vi "WriteMessage.vi"(6 "Timeout(ms)":i32, 7 "Wait for Ack? (false)":bool, 8 "error in (no error)":errorcluster, 10 "Message":T1={"Command"="", "Arguments"=variant, " Msg Id"=-1}, 11 "NetworkConnection in":refnum<class "NetworkConnection.lvclass">) -> (0 "error out":errorcluster, 2 "StillConnected?":bool, 3 "NetworkConnection out":refnum<class "NetworkConnection.lvclass">, 4 "Timed Out?":bool)   [LabVIEW 2020, in "NetworkConnection.lvclass"]
doc: "Writes a message for the Remote System. The Wait Response? input indicates wheather this method sould wait for the remote system to send a receipt confirmation response or not.\n\nJKI Network Streams Connection 1.1.1.15\nJavier Ruiz - JKI\nCopyright (c) 2020, JKI\n\nThis library is provided \"AS IS\" ,WITHOUT WARRANTIES OR CONDITIONS OF ANY KIND, either express or implied."
uses:
  NetworkConnection.lvclass
  NetworkCommand--Cluster.ctl
  NetworkMessage--Cluster.ctl
  NetworkConnection.lvclass/NetworkConnection.ctl
  Clear Errors.vi
  Random Number Within Range - I32__ogtk.vi
  <resource>/objmgr/ni.dex.rc
panel:
  # "Copyright © 2020 JKI All rights reserved.\n\nAuthor: Javier Ruiz <javier.ruiz@jki.net>\n\nThis library is provided \"AS IS\" ,WITHOUT WARRANTIES OR \nCONDITIONS OF ANY KIND, either expressed or implied.\n\nJKI -- jki.net"
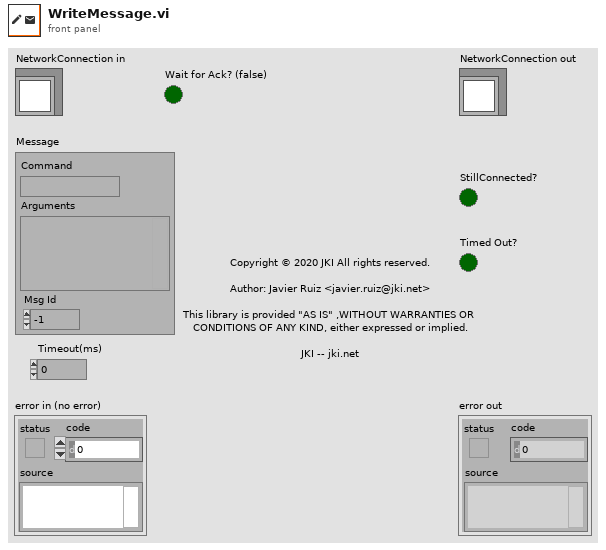
[diagram p1: front panel]
types:
  T1 = typedef "NetworkConnection.lvclass/NetworkCommand--Cluster.ctl" = cluster{"Command":string, "Arguments":variant, " Msg Id":i32}
  T2 = typedef "NetworkConnection.lvclass/NetworkMessage--Cluster.ctl" = cluster{"NetworkCommand":T1, "Wait for Ack?":bool, "Ack Id":i32}
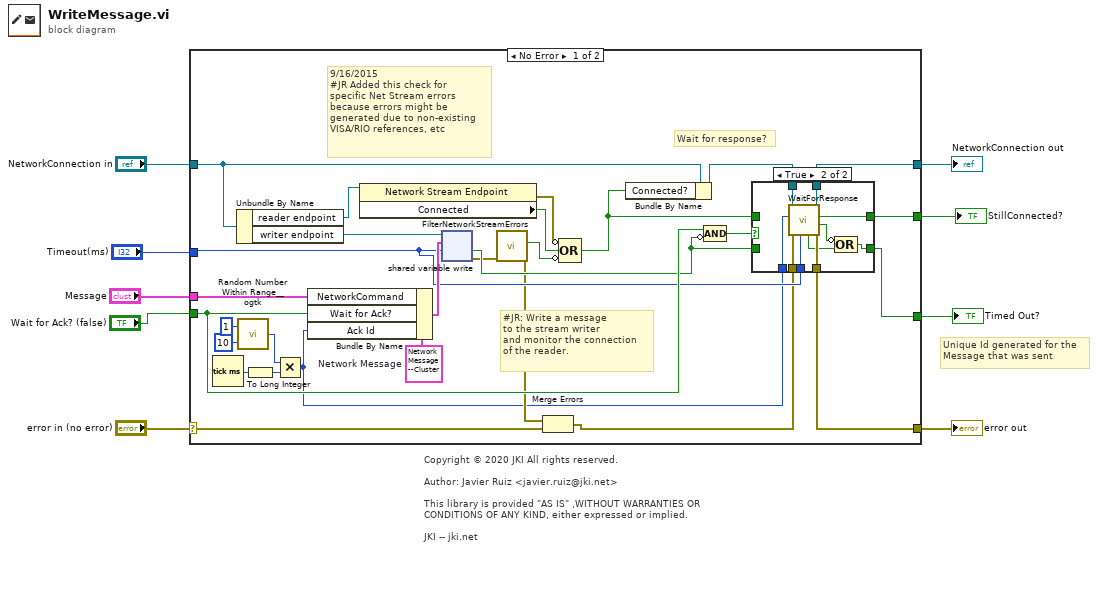
[diagram p0: block diagram]
diagram:
  # "Copyright © 2020 JKI All rights reserved.\n\nAuthor: Javier Ruiz <javier.ruiz@jki.net>\n\nThis library is provided \"AS IS\" ,WITHOUT WARRANTIES OR \nCONDITIONS OF ANY KIND, either expressed or implied.\n\nJKI -- jki.net"
  # "Unique Id generated for the\nMessage that was sent"
  n1 = case shown="No Error" "error in (no error)" {
    selector: "error in (no error)" -> [w19 w54]
    tunnel: [w29 w54] -> w8
    tunnel: [w30 w53] -> w6
    tunnel: "NetworkConnection in" -> [w36 w53]
    tunnel: "Timeout(ms)" -> [w24 _]
    tunnel: [w27 _] -> w4
    tunnel: [w23 _] -> w3
    tunnel: "Message" -> [w34 _]
    tunnel: "Wait for Ack? (false)" -> [w26 _]
    frame No Error {
      w32 = T2 {"NetworkCommand"={"Command"="", "Arguments"=variant, " Msg Id"=0}, "Wait for Ack?"=FALSE, "Ack Id"=0}  # Network Message
      # "9/16/2015\n#JR Added this check for\nspecific Net Stream errors\nbecause errors might be\ngenerated due to non-existing\nVISA/RIO references, etc"
      # "Wait for response?"
      # "#JR: Write a message\nto the stream writer\nand monitor the connection\nof the reader."
      n2 = Tick Count (ms)() -> (millisecond timer value=w11:u32)
      n3 = Unbundle By Name(w36) -> ("reader endpoint"=w38:refnum<k21>, "writer endpoint"=w35:refnum<k21>)
      n4 = call-poly "Random Number Within Range__ogtk.vi"("High"=1 ("32bit integer"), "Low"=10 ("32bit integer")) -> ("Random Number"=w14:i32)  [unwired: 3 in]
      n5 = To Long Integer(number=w11) -> (32bit integer=w15:i32)
      n6 = Multiply(x=w14, y=w15) -> (x*y=w10:i32)
      n7 = Bundle By Name(cluster=w32, "NetworkCommand"=w34, "Wait for Ack?"=w26, "Ack Id"=w10) -> (w33:T2)
      n8 = property class="Network Stream Endpoint"(reference=w38) -> (error out=w21:errorcluster, "Connected"=w37:bool)  [unwired: 1 in, 1 out]
      n9 = shared-variable-write(w35, w33, w24) -> (w20:errorcluster, w22:bool)  [unwired: 1 in, 1 out]
      n10 = call "FilterNetworkStreamErrors.vi"("error in (no error)"=w20) -> ("error out"=w17:errorcluster, "NetStream Error?"=w16:bool)  [unwired: 9 in]
      n11 = Merge Errors(w17, w19) -> (w18:errorcluster)
      n12 = Compound Arithmetic op=OR(invert w21, w37, invert w16) -> (w28:bool)
      n13 = Bundle By Name(cluster=w36, "Connected?"=w28) -> (w31:refnum<class "NetworkConnection.lvclass">)
      n14 = Compound Arithmetic op=AND(w26, invert w22) -> (w25:bool)
      n15 = case shown="True" w25 {
        tunnel: w31 -> [w42 w52]
        tunnel: [w42 w51] -> w30
        tunnel: w18 -> [w41 w50]
        tunnel: [w41 w46] -> w29
        tunnel: w28 -> [w40 _]
        tunnel: [w40 w49] -> w27
        tunnel: w10 -> [_ w48]
        tunnel: w24 -> [_ w47]
        tunnel: [w39 w43] -> w23
        tunnel: w22 -> [w39 _]
        frame False {
        }
        frame True {
          n16 = call "WaitForResponse.vi"("Timeout ms"=w47, "error in (no error)"=w50, "Ack_Id"=w48, "NetworkConnection in"=w52) -> ("error out"=w46:errorcluster, "ResponseReceived?"=w45:bool, "StillConnected?"=w49:bool, "NetworkConnection out"=w51:refnum<class "NetworkConnection.lvclass">, "Timed Out?"=w44:bool)  [unwired: 3 in]
          n17 = Compound Arithmetic op=OR(invert w45, w44) -> (w43:bool)
        }
      }
    }
    frame Error {
    }
  }
  "error out" <- w8
  "NetworkConnection out" <- w6
  "StillConnected?" <- w4
  "Timed Out?" <- w3
